vi "Receive New Subscription.vi"(8 "error in (no error)":errorcluster, 9 "Topic":string, 10 "Name":string, 11 "PubSub Status Reciever Interface in":refnum<class "PubSub Status Receiver Interface.lvclass">) -> (0 "error out":errorcluster, 3 "PubSub Status Reciever Interface out":refnum<class "PubSub Status Receiver Interface.lvclass">)   [LabVIEW 2020, in "Actor Pub Sub Channels.lvlib" / "PubSub Status Receiver Interface.lvclass"]
uses:
  PubSub Status Receiver Interface.lvclass
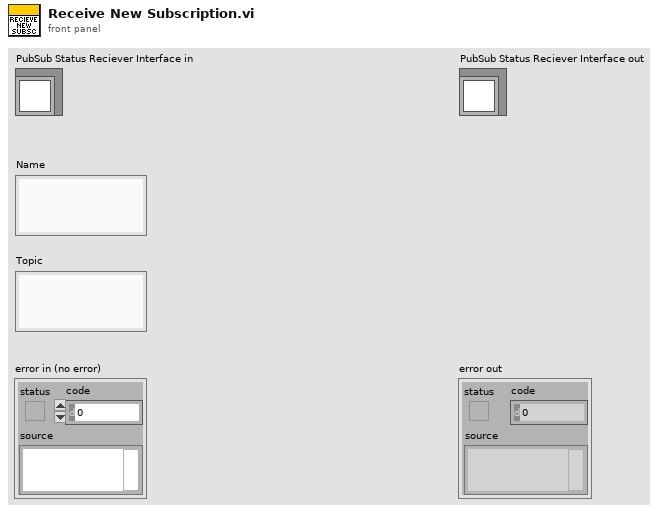
[diagram p1: front panel]
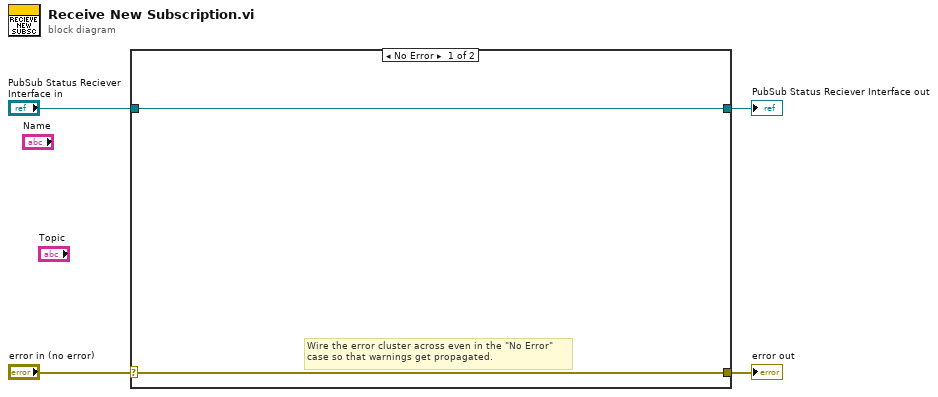
[diagram p0: block diagram]
diagram:
  n1 = case shown="No Error" "error in (no error)" {
    selector: "error in (no error)" -> [w5 w8]
    tunnel: [w5 w8] -> w3
    tunnel: [w6 w7] -> w1
    tunnel: "PubSub Status Reciever Interface in" -> [w6 w7]
    frame No Error {
      # "Wire the error cluster across even in the \"No Error\"\ncase so that warnings get propagated."
    }
    frame Error {
    }
  }
  "error out" <- w3
  "PubSub Status Reciever Interface out" <- w1
